vi "Part 1.vi"(11 "Input":string) -> (3 "Output":i64)   [LabVIEW 2021]
uses:
  <vilib>/Utility/miscctls.llb/LVMapReplaceAction.ctl
  <userlib>/_OpenG.lib/string/string.llb/Convert EOLs (String)__ogtk.vi
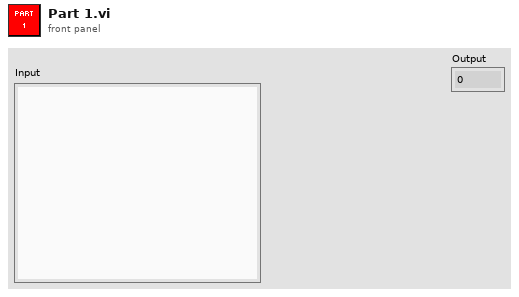
[diagram p1: front panel]
types:
  T1 = typedef "LVMapReplaceAction.ctl" = enum32{"Modify Entry only if found", "Add or Modify Entry", "Delete Entry"}
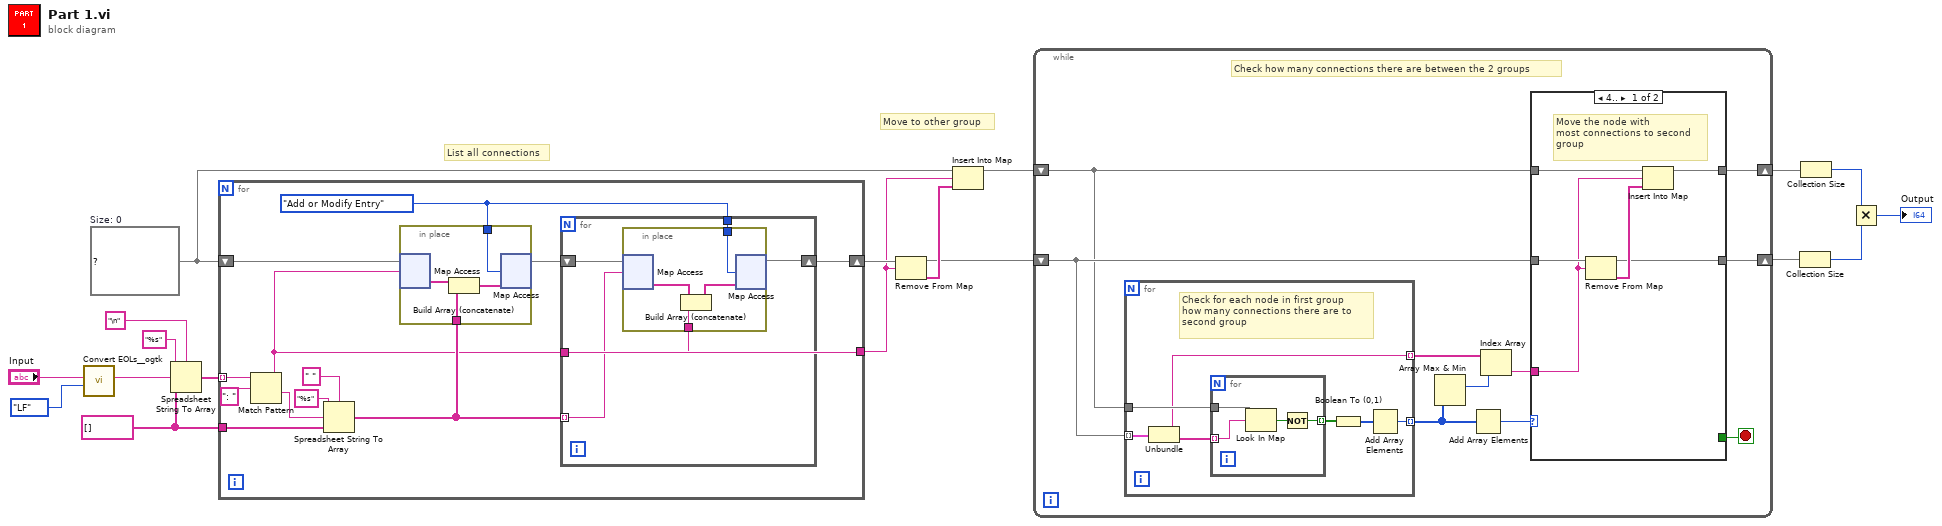
[diagram p0: block diagram]
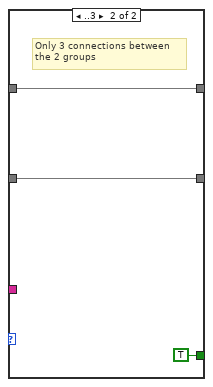
[diagram p2: hidden frame]
diagram:
  w10 = map{string, string[]} {}  # Size: 0
  w12 = string[] []
  # "Move to other group"
  # "List all connections"
  n1 = call-poly <userlib>:"Convert EOLs__ogtk.vi"("Convert to:"=enum16{"CR", "LF", "CRLF"}."LF", "String in"="Input") -> ("String out"=w16:string)  [unwired: 9 in]
  n2 = Spreadsheet String To Array(delimiter (Tab)="\n", format string="%s", spreadsheet string=w16, array type (2D Dbl)=w12) -> (array=w13:string[])
  n3 = for {
    tunnel: w13 -> [w30] mode=indexing
    tunnel: w12 -> [w28]
    shift-right: [w21] -> w11
    shift-left: w10 -> [w24]
    tunnel: [w20] -> w9
    w19 = LVMapReplaceAction."Add or Modify Entry" ("action")
    n4 = Match Pattern(string=w30, regular expression=": ") -> (before substring=w20:string, after substring=w27:string)  [unwired: 1 in, 2 out]
    n5 = Spreadsheet String To Array(delimiter (Tab)=" ", format string="%s" ("delimiter (Tab)"), spreadsheet string=w27, array type (2D Dbl)=w28) -> (array=w22:string[])
    n6 = in-place {
      in-place-border: w22 -> [w34]
      in-place-border: w19 -> [w31]
      n7 = in-place-map #1(w24, w20) -> (w32:string[])  [unwired: 1 in, 1 out]
      n8 = Build Array (concatenate)(w32, w34) -> (w33:string[])
      n9 = in-place-map #1(w33, w31) -> (w23:map{string, string[]})  [unwired: 2 out]
    }
    n10 = for {
      tunnel: w20 -> [w36]
      shift-right: [w38] -> w21
      shift-left: w23 -> [w39]
      tunnel: w22 -> [w37] mode=indexing
      tunnel: w19 -> [w35]
      n11 = in-place {
        in-place-border: w36 -> [w41]
        in-place-border: w35 -> [w40]
        n12 = in-place-map #2(w39, w37) -> (w43:string[])  [unwired: 1 in, 1 out]
        n13 = Build Array (concatenate)(w43, w41) -> (w42:string[])
        n14 = in-place-map #2(w42, w40) -> (w38:map{string, string[]})  [unwired: 2 out]
      }
    }
  }
  n15 = Remove From Map(10:w9, 11:w11) -> (1:w8:string[], 3:w7:map{string, string[]})  [unwired: 1 out]
  n16 = Insert Into Map(map in=w10, key=w9, value=w8) -> (map out=w6:map{string, string[]})  [unwired: 2 out]
  n17 = while {
    shift-right: [w51] -> w4
    shift-left: w7 -> [w50]
    shift-right: [w52] -> w5
    shift-left: w6 -> [w49]
    stop <- w53 stop-if-true
    # "Check how many connections there are between the 2 groups"
    n18 = for {
      tunnel: w50 -> [w60] mode=indexing
      tunnel: w49 -> [w58]
      tunnel: [w55] -> w46 mode=indexing
      tunnel: [w54] -> w48 mode=indexing
      # "Check for each node in first group\nhow many connections there are to \nsecond group"
      n19 = Unbundle(w60) -> (w54:string, w59:string[])
      n20 = for {
        tunnel: w59 -> [w63] mode=indexing
        tunnel: w58 -> [w64]
        tunnel: [w61] -> w57 mode=indexing
        n21 = Look In Map(map=w64, key=w63) -> (key not found?=w62:bool)  [unwired: 1 in, 1 out]
        n22 = Not(x=w62) -> (.not. x?=w61:bool)
      }
      n23 = Boolean To (0,1)(Boolean=w57) -> (0, 1=w56:i16[])
      n24 = Add Array Elements(numeric array=w56) -> (sum=w55:i16)
    }
    n25 = Array Max & Min(array=w46) -> (max index (indices)=w47:i32)  [unwired: 3 out]
    n26 = Add Array Elements(numeric array=w46) -> (sum=w45:i16)
    n27 = Index Array(array=w48, index=w47) -> (element=w44:string)
    n28 = case shown="4.." w45 {
      tunnel: [_ TRUE] -> w53
      tunnel: w49 -> [w69 w72]
      tunnel: [w66 w72] -> w52
      tunnel: w50 -> [w68 w71]
      tunnel: [w65 w71] -> w51
      tunnel: w44 -> [w67 _]
      frame 4.. {
        # "Move the node with\nmost connections to second\ngroup"
        n29 = Remove From Map(10:w67, 11:w68) -> (1:w70:string[], 3:w65:map{string, string[]})  [unwired: 1 out]
        n30 = Insert Into Map(map in=w69, key=w67, value=w70) -> (map out=w66:map{string, string[]})  [unwired: 2 out]
      }
      frame ..3 {
        # "Only 3 connections between\nthe 2 groups"
      }
    }
  }
  n31 = Collection Size(1:w4) -> (0:w3:i32)
  n32 = Collection Size(1:w5) -> (0:w2:i32)
  n33 = Multiply(x=w2, y=w3) -> (x*y=→"Output":i32)
